vi "setSetpoint.vi"(0 "FlowControlActuator in":refnum<class "PressureServoActuatorClosed.lvclass">, 5 "ILC in":refnum<class "ILC.lvclass">, 7 "Force Setpoint":dbl[unit], 9 "Measured Force":dbl[unit], 11 "error in (no error)":errorcluster) -> (4 "FlowControlActuator out":refnum<class "PressureServoActuatorClosed.lvclass">, 6 "ILC out":refnum<class "ILC.lvclass">, 15 "error out":errorcluster)   [LabVIEW 2015, in "PressureServoActuatorClosed.lvclass"]
uses:
  PressureServoActuatorClosed.lvclass
  <userlib>/Common/ILC/ILC/ILC.lvclass
  PressureServoActuatorClosed.lvclass/PressureServoActuatorClosed.ctl
  <vilib>/addons/control/pid/pid.llb/PID (DBL).vi
  ActuatorCylinder/IActuatorCylinder/IActuatorCylinder.lvclass
  Calculators/ForceToPressureServoVoltage/ForceToPressureServoVoltage.lvclass
  <vilib>/addons/control/pid/NI_PID_pid.lvlib
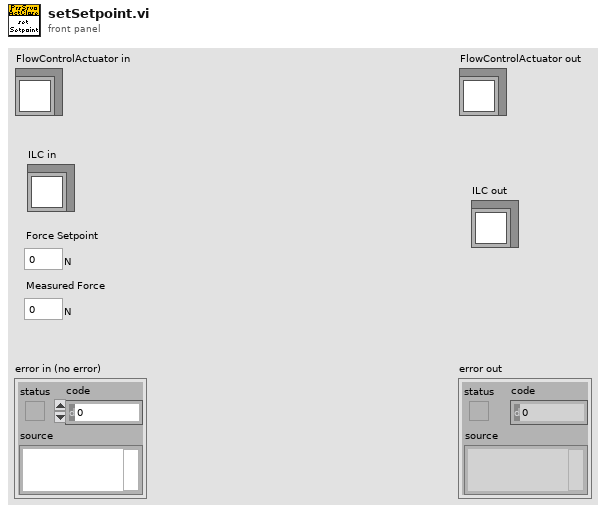
[diagram p1: front panel]
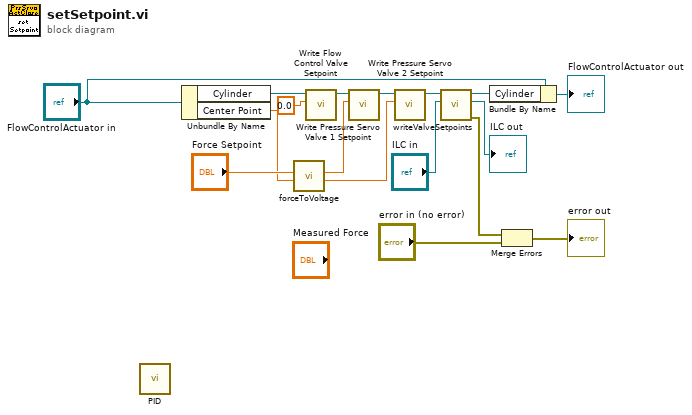
[diagram p0: block diagram]
diagram:
  n1 = call-poly <vilib>:"PID.vi"() -> ()  [unwired: 10 in, 2 out]
  n2 = Unbundle By Name("FlowControlActuator in") -> ("Cylinder"=w10:refnum<class "IActuatorCylinder.lvclass">, "Center Point"=w3:dbl[unit])
  n3 = call "forceToVoltage.vi"("Center Point"=w3, "Force"="Force Setpoint") -> ("Voltage 2"=w1:dbl[unit], "Voltage 1"=w2:dbl[unit])  [unwired: 6 in, 2 out]
  n4 = call-dynamic "Write Flow Control Valve Setpoint.vi"("Flow Control Valve Setpoint"=dbl[unit] 0.0, "IActuatorCylinder in"=w10) -> ("IActuatorCylinder out"=w9:refnum<class "IActuatorCylinder.lvclass">)  [unwired: 9 in]
  n5 = call-dynamic "Write Pressure Servo Valve 1 Setpoint.vi"("Pressure Servo Valve 1 Setpoint"=w2, "IActuatorCylinder in"=w9) -> ("IActuatorCylinder out"=w8:refnum<class "IActuatorCylinder.lvclass">)  [unwired: 9 in]
  n6 = call-dynamic "Write Pressure Servo Valve 2 Setpoint.vi"("Pressure Servo Valve 2 Setpoint"=w1, "IActuatorCylinder in"=w8) -> ("IActuatorCylinder out"=w11:refnum<class "IActuatorCylinder.lvclass">)  [unwired: 9 in]
  n7 = call-dynamic "writeValveSetpoints.vi"("ILC in"="ILC in", "IActuatorCylinder in"=w11) -> ("error out"=w15:errorcluster, "ILC out"=→"ILC out":refnum<class "ILC.lvclass">, "IActuatorCylinder out"=w12:refnum<class "IActuatorCylinder.lvclass">)  [unwired: 7 in]
  n8 = Bundle By Name(cluster="FlowControlActuator in", "Cylinder"=w12) -> (→"FlowControlActuator out":refnum<class "PressureServoActuatorClosed.lvclass">)
  n9 = Merge Errors(w15, "error in (no error)") -> (→"error out":errorcluster)
